vi "Colaborativo_Dídier Javier Ramírez Henao.vi"() -> ()   [LabVIEW 2020]
uses:
  <vilib>/Instr/_visa.llb/VISA Configure Serial Port (Instr).vi
panel:
  out "Nivel":dbl
  out "read buffer":string
  out "Mezclado":bool
  out "ABORTAR":bool
  out "Parada":bool
  out "Marcha":bool
  out "AspaBoolean":bool
  out "NivelB":bool
  out "NivelM":bool
  out "NivelA":bool
  in  "VISA resource name":refnum<visa-resource-name>
  out "NIVEL":dbl(slide) scale=0.0..50.0 scale format="%#.2g"
  in  "Abortar":bool
  in  "Parada 3":bool
  in  "Marcha 3":bool
  out "Inicio":bool
  out "Fin":bool
  # "Chocolate"
  # "Azúcar"
  # "Dídier Javier Ramírez Henao"
  # "Mezclado"
  # "Nivel alto"
  # "Mezclado"
  # "Nivel medio"
  # "Subproceso 3 _ Mezclado"
  # "Nivel bajo"
  # "Fin"
  # "Pulsadores de mando"
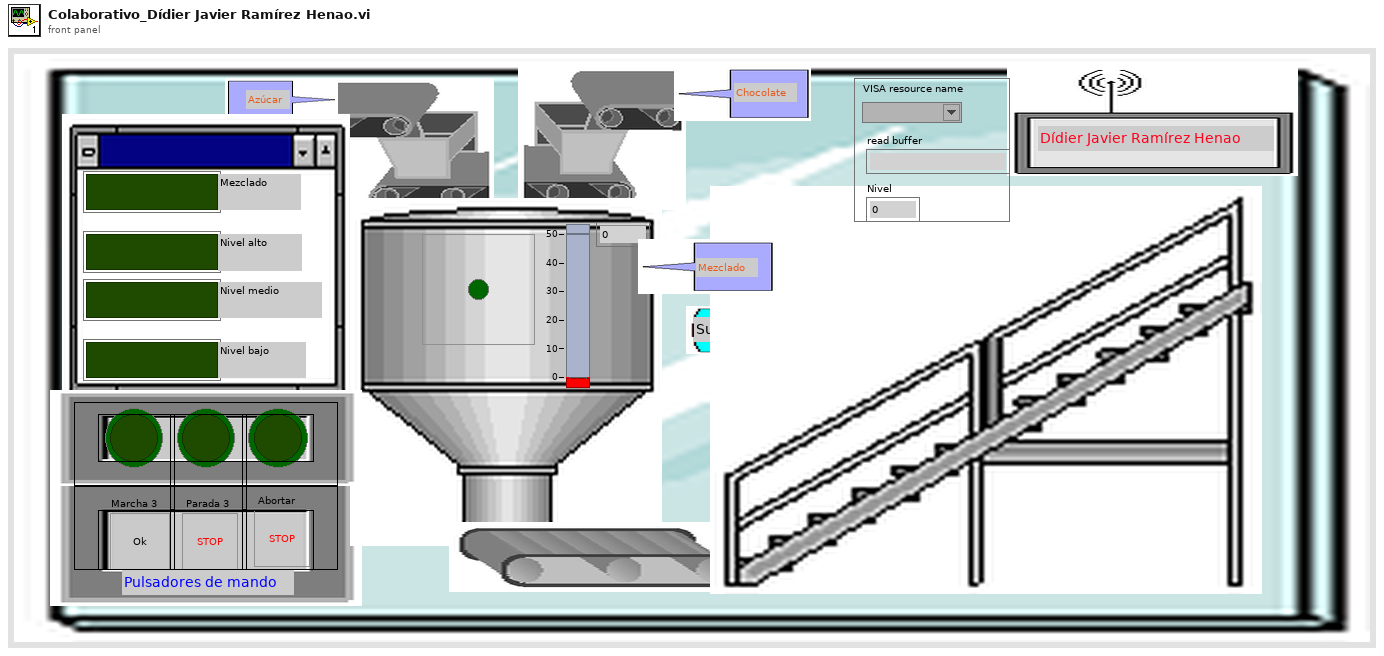
[diagram p1: front panel]
types:
  T1 = enum16{"INICIO", "NIVELA", "NIVELB", "NIVELM", "MEZCLADO", "PARO", "ABORTAR", "FIN"}
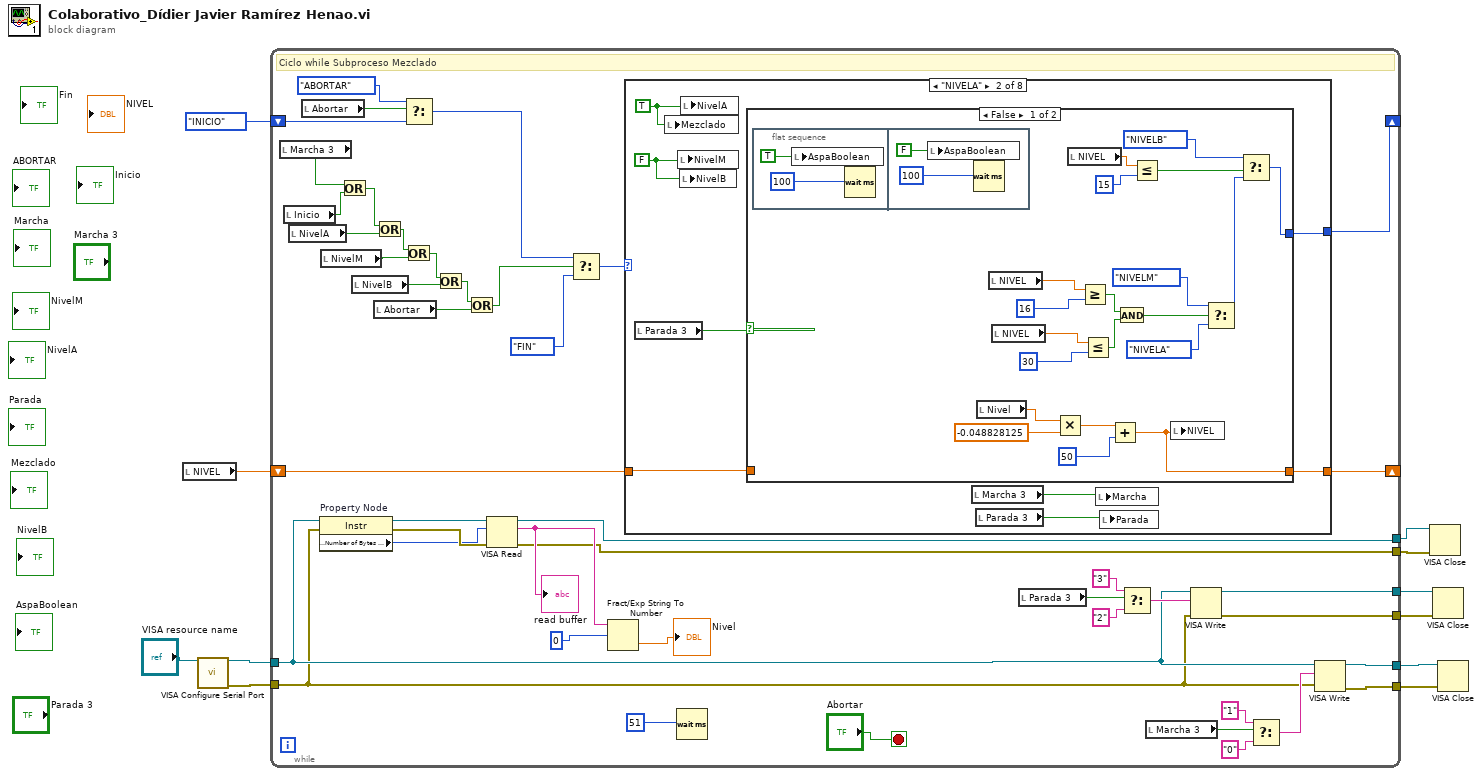
[diagram p0: block diagram]
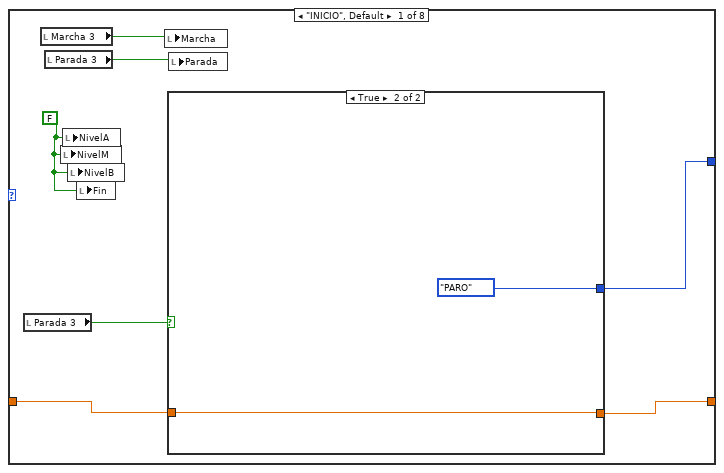
[diagram p2: hidden frame]
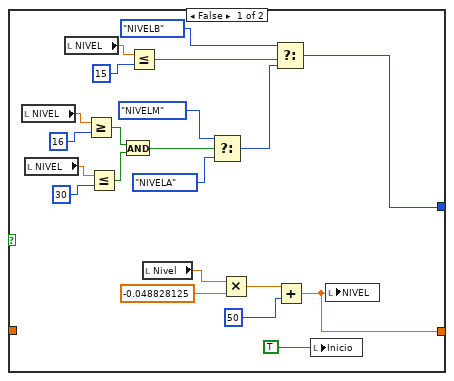
[diagram p3: hidden frame]
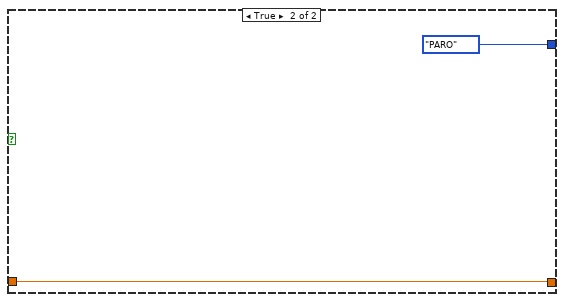
[diagram p4: hidden frame]
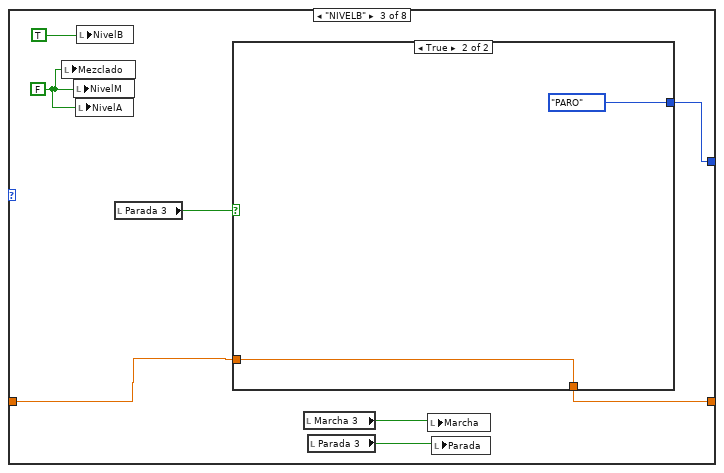
[diagram p5: hidden frame]
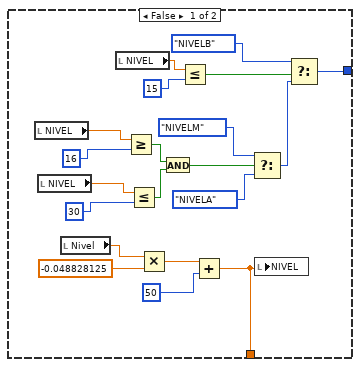
[diagram p6: hidden frame]
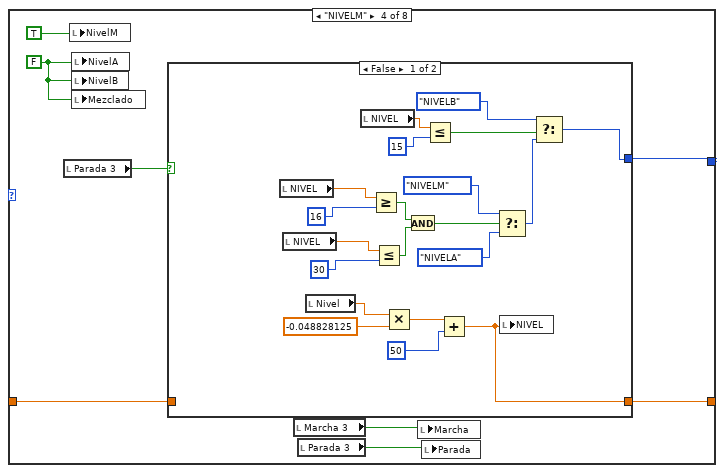
[diagram p7: hidden frame]
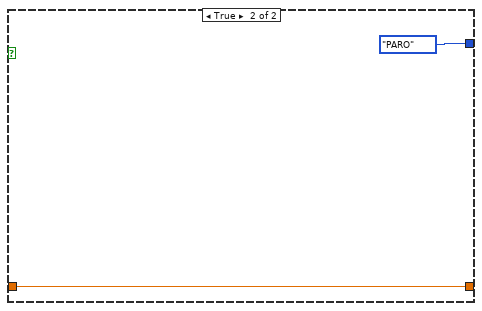
[diagram p8: hidden frame]
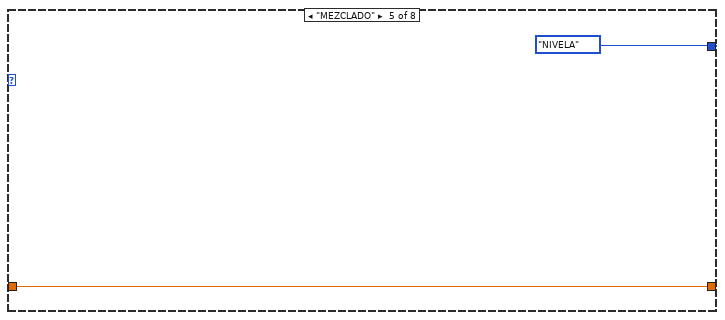
[diagram p9: hidden frame]
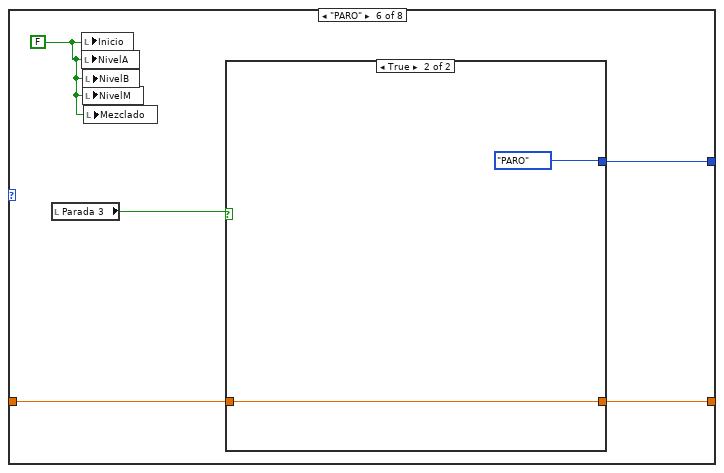
[diagram p10: hidden frame]
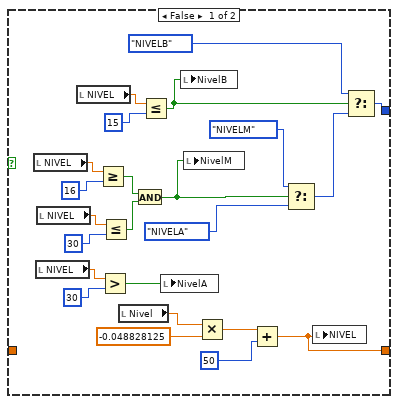
[diagram p11: hidden frame]
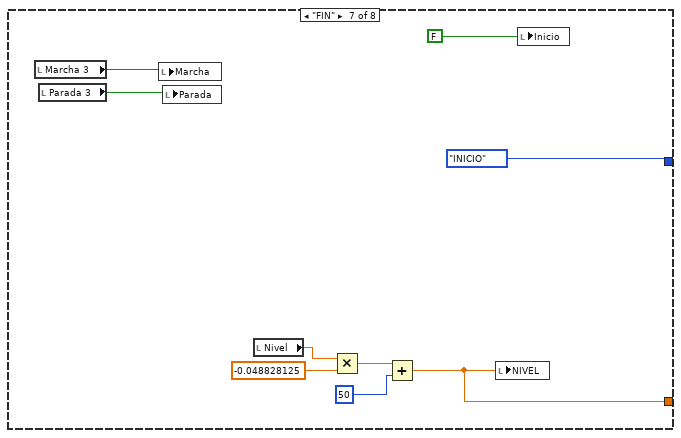
[diagram p12: hidden frame]
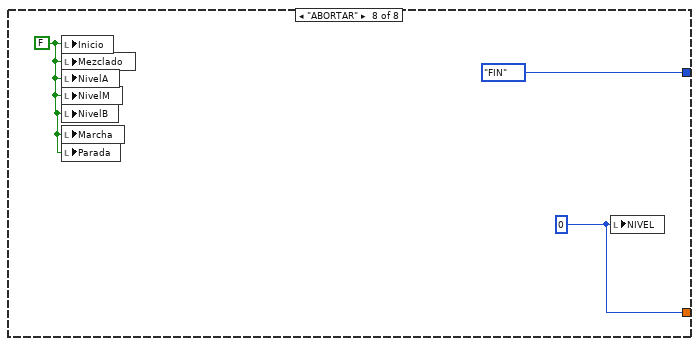
[diagram p13: hidden frame]
diagram:
  n1 = local read "NIVEL"() -> (w3:dbl)
  n2 = call-poly "VISA Configure Serial Port"("VISA resource name"="VISA resource name") -> ("VISA resource name out"=w9:refnum<visa-resource-name>, "error out"=w8:errorcluster)  [unwired: 13 in]
  n3 = while {
    shift-right: [w43] -> _
    shift-left: T1."INICIO" -> [w55]
    shift-right: [w38] -> _
    shift-left: w3 -> [w39]
    tunnel: w9 -> [w18]
    tunnel: w8 -> [w17]
    tunnel: [w37] -> w7
    tunnel: [w36] -> w6
    tunnel: [w26] -> w5
    tunnel: [w25] -> w4
    tunnel: [w16] -> w2
    tunnel: [w15] -> w1
    stop <- "Abortar" stop-if-true
    # "Ciclo while Subproceso Mezclado"
    n4 = local read "Marcha 3"() -> (w14:bool)
    n5 = local read "Inicio"() -> (w52:bool)
    n6 = local read "NivelA"() -> (w50:bool)
    n7 = local read "Abortar"() -> (w45:bool)
    n8 = property on="Property Node" class="Instr"(reference=w18, error in=w17) -> (reference out=w30:refnum<visa-resource-name>, error out=w29:errorcluster, "Serial Settings:Number of Bytes at Serial Port"=w28:u32)
    n9 = local read "NivelM"() -> (w48:bool)
    n10 = Or(x=w14, y=w52) -> (x .or. y?=w51:bool)
    n11 = local read "NivelB"() -> (w46:bool)
    n12 = local read "Abortar"() -> (w13:bool)
    n13 = Or(x=w51, y=w50) -> (x .or. y?=w49:bool)
    n14 = Select(t=T1."ABORTAR", s=w45, f=w55) -> (s? t:f=w53:T1)
    n15 = Or(x=w49, y=w48) -> (x .or. y?=w47:bool)
    n16 = Or(x=w47, y=w46) -> (x .or. y?=w44:bool)
    n17 = Or(x=w44, y=w13) -> (x .or. y?=w12:bool)
    n18 = VISA Read(VISA resource name=w30, byte count=w28, error in (no error)=w29) -> (VISA resource name out=w26:refnum<visa-resource-name>, read buffer=w27:string, error out=w25:errorcluster)  [unwired: 1 out]
    "read buffer" <- w27
    n19 = Select(t=w53, s=w12, f=T1."FIN") -> (s? t:f=w40:T1)
    n20 = Fract/Exp String To Number(string=w27, offset=0) -> (number=→"Nivel":dbl)  [unwired: 2 in, 1 out]
    n21 = case shown="\"NIVELA\"" w40 {
      tunnel: [w60 w92 w123 w157 T1."NIVELA" w184 T1."INICIO" T1."FIN"] -> w43
      tunnel: w39 -> [w56 w90 w121 w151 w180 w183 _ _]
      tunnel: [w59 w89 w120 w150 w180 w182 w215 w221] -> w38
      frame "INICIO", Default {
        w62 = FALSE
        n22 = local read "Parada 3"() -> (w61:bool)
        n23 = local read "Marcha 3"() -> (w58:bool)
        n24 = local read "Parada 3"() -> (w57:bool)
        n25 = local write "NivelM"(w62) -> ()
        n26 = local write "NivelA"(w62) -> ()
        n27 = local write "NivelB"(w62) -> ()
        n28 = local write "Fin"(w62) -> ()
        n29 = local write "Marcha"(w58) -> ()
        n30 = case shown="True" w61 {
          tunnel: [w64 T1."PARO"] -> w60
          tunnel: [w63 w84] -> w59
          tunnel: w56 -> [_ w84]
          frame False {
            n31 = local read "NIVEL"() -> (w74:dbl)
            n32 = local read "NIVEL"() -> (w73:dbl)
            n33 = local read "NIVEL"() -> (w77:dbl)
            n34 = Greater Or Equal?(x=w74, y=16) -> (x >= y?=w71:bool)
            n35 = Less Or Equal?(x=w73, y=30) -> (x <= y?=w69:bool)
            n36 = And(x=w71, y=w69) -> (x .and. y?=w68:bool)
            n37 = Less Or Equal?(x=w77, y=15) -> (x <= y?=w76:bool)
            n38 = local read "Nivel"() -> (w81:dbl)
            n39 = Select(t=T1."NIVELM", s=w68, f=T1."NIVELA") -> (s? t:f=w65:T1)
            n40 = Multiply(x=w81, y=-0.048828125) -> (x*y=w82:dbl)
            n41 = Select(t=T1."NIVELB", s=w76, f=w65) -> (s? t:f=w64:T1)
            n42 = Add(x=w82, y=50) -> (x+y=w63:dbl)
            n43 = local write "Inicio"(TRUE) -> ()
            n44 = local write "NIVEL"(w63) -> ()
          }
          frame True {
          }
        }
        n45 = local write "Parada"(w57) -> ()
      }
      frame "NIVELA" {
        w91 = FALSE
        w86 = TRUE
        n46 = local read "Parada 3"() -> (w93:bool)
        n47 = local write "Mezclado"(w86) -> ()
        n48 = local write "NivelM"(w91) -> ()
        n49 = local write "NivelB"(w91) -> ()
        n50 = local write "NivelA"(w86) -> ()
        n51 = case shown="False" w93 {
          tunnel: [w99 T1."PARO"] -> w92
          tunnel: w90 -> [_ w118]
          tunnel: [w94 w118] -> w89
          frame False {
            n52 = flat-sequence {
              frame #0 {
                n53 = local write "AspaBoolean"(TRUE) -> ()
                n54 = Wait (ms)(milliseconds to wait=100) -> ()  [unwired: 1 out]
              }
              frame #1 {
                n55 = local write "AspaBoolean"(FALSE) -> ()
                n56 = Wait (ms)(milliseconds to wait=100) -> ()  [unwired: 1 out]
              }
            }
            n57 = local read "Nivel"() -> (w97:dbl)
            n58 = local read "NIVEL"() -> (w111:dbl)
            n59 = local read "NIVEL"() -> (w110:dbl)
            n60 = Multiply(x=w97, y=-0.048828125) -> (x*y=w98:dbl)
            n61 = local read "NIVEL"() -> (w113:dbl)
            n62 = Greater Or Equal?(x=w111, y=16) -> (x >= y?=w109:bool)
            n63 = Less Or Equal?(x=w110, y=30) -> (x <= y?=w108:bool)
            n64 = Add(x=w98, y=50) -> (x+y=w94:dbl)
            n65 = And(x=w109, y=w108) -> (x .and. y?=w107:bool)
            n66 = Less Or Equal?(x=w113, y=15) -> (x <= y?=w112:bool)
            n67 = local write "NIVEL"(w94) -> ()
            n68 = Select(t=T1."NIVELM", s=w107, f=T1."NIVELA") -> (s? t:f=w106:T1)
            n69 = Select(t=T1."NIVELB", s=w112, f=w106) -> (s? t:f=w99:T1)
          }
          frame True {
          }
        }
        n70 = local read "Marcha 3"() -> (w88:bool)
        n71 = local read "Parada 3"() -> (w87:bool)
        n72 = local write "Marcha"(w88) -> ()
        n73 = local write "Parada"(w87) -> ()
      }
      frame "NIVELB" {
        w126 = FALSE
        n74 = local write "Mezclado"(w126) -> ()
        n75 = local write "NivelM"(w126) -> ()
        n76 = local write "NivelA"(w126) -> ()
        n77 = local write "NivelB"(TRUE) -> ()
        n78 = local read "Parada 3"() -> (w122:bool)
        n79 = case shown="True" w122 {
          tunnel: [w129 T1."PARO"] -> w123
          tunnel: w121 -> [_ w148]
          tunnel: [w128 w148] -> w120
          frame False {
            n80 = local read "NIVEL"() -> (w145:dbl)
            n81 = local read "NIVEL"() -> (w144:dbl)
            n82 = local read "Nivel"() -> (w138:dbl)
            n83 = local read "NIVEL"() -> (w147:dbl)
            n84 = Greater Or Equal?(x=w145, y=16) -> (x >= y?=w143:bool)
            n85 = Less Or Equal?(x=w144, y=30) -> (x <= y?=w142:bool)
            n86 = Multiply(x=w138, y=-0.048828125) -> (x*y=w139:dbl)
            n87 = And(x=w143, y=w142) -> (x .and. y?=w141:bool)
            n88 = Less Or Equal?(x=w147, y=15) -> (x <= y?=w146:bool)
            n89 = Add(x=w139, y=50) -> (x+y=w128:dbl)
            n90 = Select(t=T1."NIVELM", s=w141, f=T1."NIVELA") -> (s? t:f=w140:T1)
            n91 = local write "NIVEL"(w128) -> ()
            n92 = Select(t=T1."NIVELB", s=w146, f=w140) -> (s? t:f=w129:T1)
          }
          frame True {
          }
        }
        n93 = local read "Marcha 3"() -> (w125:bool)
        n94 = local read "Parada 3"() -> (w124:bool)
        n95 = local write "Marcha"(w125) -> ()
        n96 = local write "Parada"(w124) -> ()
      }
      frame "NIVELM" {
        w152 = FALSE
        n97 = local read "Parada 3"() -> (w156:bool)
        n98 = local write "NivelM"(TRUE) -> ()
        n99 = local write "NivelA"(w152) -> ()
        n100 = local write "NivelB"(w152) -> ()
        n101 = local write "Mezclado"(w152) -> ()
        n102 = case shown="False" w156 {
          tunnel: [w163 T1."PARO"] -> w157
          tunnel: w151 -> [_ w178]
          tunnel: [w158 w178] -> w150
          frame False {
            n103 = local read "NIVEL"() -> (w173:dbl)
            n104 = local read "NIVEL"() -> (w172:dbl)
            n105 = local read "Nivel"() -> (w161:dbl)
            n106 = local read "NIVEL"() -> (w177:dbl)
            n107 = Greater Or Equal?(x=w173, y=16) -> (x >= y?=w171:bool)
            n108 = Less Or Equal?(x=w172, y=30) -> (x <= y?=w170:bool)
            n109 = Multiply(x=w161, y=-0.048828125) -> (x*y=w162:dbl)
            n110 = And(x=w171, y=w170) -> (x .and. y?=w169:bool)
            n111 = Less Or Equal?(x=w177, y=15) -> (x <= y?=w176:bool)
            n112 = Add(x=w162, y=50) -> (x+y=w158:dbl)
            n113 = Select(t=T1."NIVELM", s=w169, f=T1."NIVELA") -> (s? t:f=w164:T1)
            n114 = local write "NIVEL"(w158) -> ()
            n115 = Select(t=T1."NIVELB", s=w176, f=w164) -> (s? t:f=w163:T1)
          }
          frame True {
          }
        }
        n116 = local read "Marcha 3"() -> (w155:bool)
        n117 = local read "Parada 3"() -> (w154:bool)
        n118 = local write "Marcha"(w155) -> ()
        n119 = local write "Parada"(w154) -> ()
      }
      frame "MEZCLADO" {
      }
      frame "PARO" {
        w186 = FALSE
        n120 = local read "Parada 3"() -> (w185:bool)
        n121 = local write "Inicio"(w186) -> ()
        n122 = local write "NivelA"(w186) -> ()
        n123 = local write "NivelB"(w186) -> ()
        n124 = local write "NivelM"(w186) -> ()
        n125 = local write "Mezclado"(w186) -> ()
        n126 = case shown="True" w185 {
          tunnel: [w195 T1."PARO"] -> w184
          tunnel: w183 -> [_ w210]
          tunnel: [w187 w210] -> w182
          frame False {
            n127 = local read "NIVEL"() -> (w208:dbl)
            n128 = local read "NIVEL"() -> (w201:dbl)
            n129 = local read "NIVEL"() -> (w207:dbl)
            n130 = local read "NIVEL"() -> (w209:dbl)
            n131 = Greater Or Equal?(x=w208, y=16) -> (x >= y?=w206:bool)
            n132 = Greater?(x=w201, y=30) -> (0:w200:bool)
            n133 = Less Or Equal?(x=w207, y=30) -> (x <= y?=w205:bool)
            n134 = local read "Nivel"() -> (w190:dbl)
            n135 = And(x=w206, y=w205) -> (x .and. y?=w202:bool)
            n136 = Less Or Equal?(x=w209, y=15) -> (x <= y?=w203:bool)
            n137 = local write "NivelA"(w200) -> ()
            n138 = local write "NivelB"(w203) -> ()
            n139 = local write "NivelM"(w202) -> ()
            n140 = Multiply(x=w190, y=-0.048828125) -> (x*y=w191:dbl)
            n141 = Add(x=w191, y=50) -> (x+y=w187:dbl)
            n142 = Select(t=T1."NIVELM", s=w202, f=T1."NIVELA") -> (s? t:f=w204:T1)
            n143 = local write "NIVEL"(w187) -> ()
            n144 = Select(t=T1."NIVELB", s=w203, f=w204) -> (s? t:f=w195:T1)
          }
          frame True {
          }
        }
      }
      frame "FIN" {
        n145 = local read "Marcha 3"() -> (w214:bool)
        n146 = local read "Parada 3"() -> (w213:bool)
        n147 = local write "Marcha"(w214) -> ()
        n148 = local write "Parada"(w213) -> ()
        n149 = local read "Nivel"() -> (w219:dbl)
        n150 = Multiply(x=w219, y=-0.048828125) -> (x*y=w218:dbl)
        n151 = Add(x=w218, y=50) -> (x+y=w215:dbl)
        n152 = local write "NIVEL"(w215) -> ()
        n153 = local write "Inicio"(FALSE) -> ()
      }
      frame "ABORTAR" {
        w221 = 0
        w222 = FALSE
        n154 = local write "Inicio"(w222) -> ()
        n155 = local write "Mezclado"(w222) -> ()
        n156 = local write "NivelA"(w222) -> ()
        n157 = local write "NivelM"(w222) -> ()
        n158 = local write "NivelB"(w222) -> ()
        n159 = local write "Marcha"(w222) -> ()
        n160 = local write "Parada"(w222) -> ()
        n161 = local write "NIVEL"(w221) -> ()
      }
    }
    n162 = Wait (ms)(milliseconds to wait=51) -> ()  [unwired: 1 out]
    n163 = local read "Parada 3"() -> (w20:bool)
    n164 = Select(t="3", s=w20, f="2") -> (s? t:f=w19:string)
    n165 = local read "Marcha 3"() -> (w34:bool)
    n166 = VISA Write(VISA resource name=w18, write buffer=w19, error in (no error)=w17) -> (VISA resource name out=w16:refnum<visa-resource-name>, error out=w15:errorcluster)  [unwired: 1 out]
    n167 = Select(t="1", s=w34, f="0") -> (s? t:f=w31:string)
    n168 = VISA Write(VISA resource name=w18, write buffer=w31, error in (no error)=w17) -> (VISA resource name out=w37:refnum<visa-resource-name>, error out=w36:errorcluster)  [unwired: 1 out]
  }
  n169 = VISA Close(VISA resource name=w5, error in (no error)=w4) -> ()  [unwired: 1 out]
  n170 = VISA Close(VISA resource name=w2, error in (no error)=w1) -> ()  [unwired: 1 out]
  n171 = VISA Close(VISA resource name=w7, error in (no error)=w6) -> ()  [unwired: 1 out]
